vi "DataPacker_Wait.vi"(8 "error in (no error)":errorcluster, 11 "DataPacker in":refnum<class "DataPacker.lvclass">) -> (0 "error out":errorcluster, 2 "% Time Packing (Serializing Queued Data)":dbl, 3 "DataPacker out":refnum<class "DataPacker.lvclass">)   [LabVIEW 2018, in "feGEM DataPacker.lvlib" / "DataPacker.lvclass"]
uses:
  DataPacker.lvclass
  DataPacker.lvclass/DataPacker.ctl
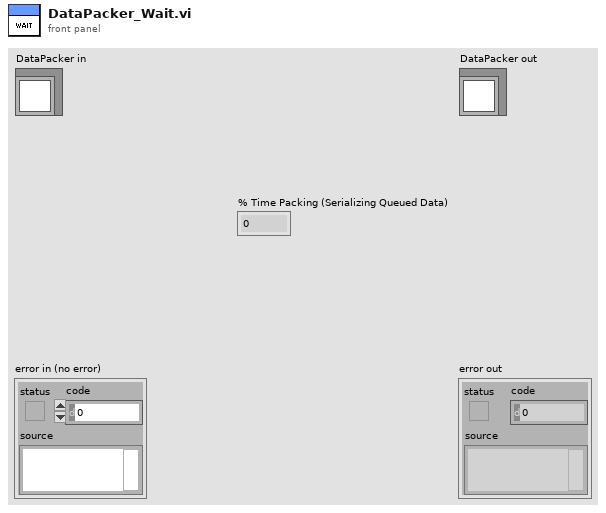
[diagram p1: front panel]
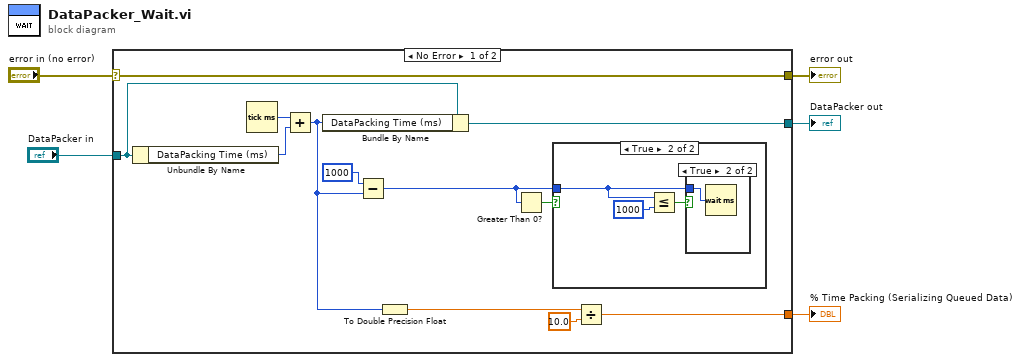
[diagram p0: block diagram]
diagram:
  n1 = case shown="No Error" "error in (no error)" {
    selector: "error in (no error)" -> [w17 w23]
    tunnel: [w17 w23] -> w4
    tunnel: [w10 w22] -> w2
    tunnel: "DataPacker in" -> [w11 w22]
    tunnel: [w6 _] -> w1
    frame No Error {
      n2 = Unbundle By Name(w11) -> ("DataPacking Time (ms)"=w14:u32)
      n3 = Tick Count (ms)() -> (millisecond timer value=w16:u32)
      n4 = Add(x=w16, y=w14) -> (x+y=w9:u32)
      n5 = Bundle By Name(cluster=w11, "DataPacking Time (ms)"=w9) -> (w10:refnum<class "DataPacker.lvclass">)
      n6 = Subtract(x=u32 1000, y=w9) -> (x-y=w12:u32)
      n7 = To Double Precision Float(number=w9) -> (double precision float=w8:dbl)
      n8 = Greater Than 0?(x=w12) -> (x > 0?=w13:bool)
      n9 = case shown="True" w13 {
        tunnel: w12 -> [_ w20]
        frame False {
        }
        frame True {
          n10 = Less Or Equal?(x=w20, y=u32 1000) -> (x <= y?=w18:bool)
          n11 = case shown="True" w18 {
            tunnel: w20 -> [_ w21]
            frame False {
            }
            frame True {
              n12 = Wait (ms)(milliseconds to wait=w21) -> ()  [unwired: 1 out]
            }
          }
        }
      }
      n13 = Divide(x=w8, y=10.0) -> (x/y=w6:dbl)
    }
    frame Error {
    }
  }
  "error out" <- w4
  "DataPacker out" <- w2
  "% Time Packing (Serializing Queued Data)" <- w1
